vi "In Compliance Query.vi"(8 "error in (no error)":errorcluster, 11 "VISA resource name":refnum<visa-resource-name>) -> (0 "error out":errorcluster, 1 "Current Source":bool, 2 "Voltage Source":bool, 3 "VISA resource name out":refnum<visa-resource-name>)   [LabVIEW 2020, in "Keithley 2450.lvlib"]
doc: "Queries the instrument to determine if source is in current or voltage compliance."
uses:
  <instrlib>/Keithley 2450/Keithley 2450.lvlib
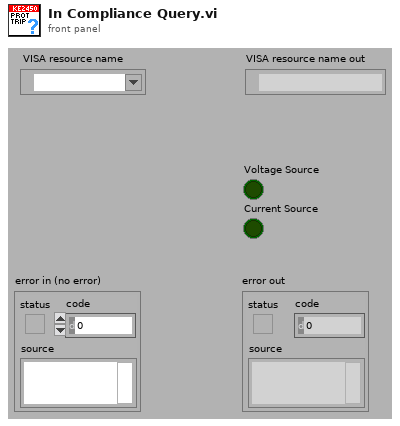
[diagram p1: front panel]
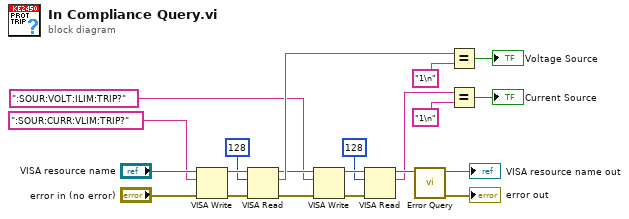
[diagram p0: block diagram]
diagram:
  n1 = VISA Write(VISA resource name="VISA resource name", write buffer=":SOUR:CURR:VLIM:TRIP?" ("f"), error in (no error)="error in (no error)") -> (VISA resource name out=w16:refnum<visa-resource-name>, error out=w17:errorcluster)  [unwired: 1 out]
  n2 = VISA Read(VISA resource name=w16, byte count=u32 128, error in (no error)=w17) -> (VISA resource name out=w6:refnum<visa-resource-name>, read buffer=w15:string, error out=w7:errorcluster)  [unwired: 1 out]
  n3 = VISA Write(VISA resource name=w6, write buffer=":SOUR:VOLT:ILIM:TRIP?", error in (no error)=w7) -> (VISA resource name out=w9:refnum<visa-resource-name>, error out=w10:errorcluster)  [unwired: 1 out]
  n4 = VISA Read(VISA resource name=w9, byte count=u32 128, error in (no error)=w10) -> (VISA resource name out=w5:refnum<visa-resource-name>, read buffer=w1:string)  [unwired: 2 out]
  n5 = call <instrlib>:"Error Query.vi"("VISA resource name"=w5) -> ("error out"=→"error out":errorcluster, "VISA resource name out"=→"VISA resource name out":refnum<visa-resource-name>)  [unwired: 1 in, 8 out]
  n6 = Equal?(x=w15, y="1\n") -> (x = y?=→"Voltage Source":bool)
  n7 = Equal?(x=w1, y="1\n") -> (x = y?=→"Current Source":bool)
